vi "Galvo status.vi"() -> ()   [LabVIEW 2018]
uses:
  Controls/ScanType.ctl
  Controls/FGV Actions.ctl
panel:
  out "Scan Type [Out]":T1
  out "Error Out":errorcluster
  in  "Error In":errorcluster
  in  "Actions":T2=enum."Clear"
  out "Status Out":bool
  in  "Status In":bool
  in  "Scan Type [In]":T1
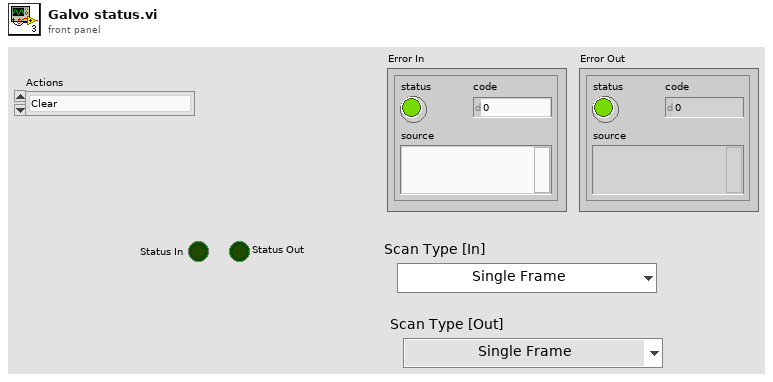
[diagram p1: front panel]
types:
  T1 = typedef "ScanType.ctl" = enum16{"Single Frame", "Continuous Frame", "ROI Line", "Vibratome", "Mosaic", "Mosaic + Slice"}
  T2 = typedef "FGV Actions.ctl" = enum16{"Init", "Set", "Get", "Clear"}
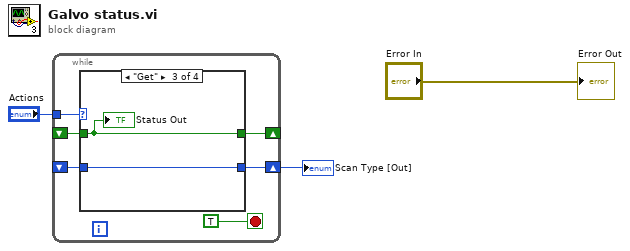
[diagram p0: block diagram]
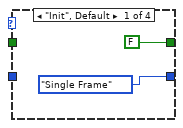
[diagram p2: hidden frame]
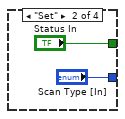
[diagram p3: hidden frame]
diagram:
  n1 = while {
    tunnel: "Actions" -> [w8]
    shift-right: [w7] -> _
    shift-left: _ -> [w6]
    shift-right: [w5] -> w1
    shift-left: _ -> [w4]
    stop <- TRUE stop-if-true
    n2 = case shown="\"Get\"" w8 {
      tunnel: [FALSE "Status In" w15 _] -> w7
      tunnel: w6 -> [_ _ w15 _]
      tunnel: [ScanType."Single Frame" ("Scan Type") "Scan Type [In]" w14 _] -> w5
      tunnel: w4 -> [_ _ w14 _]
      frame "Init", Default {
      }
      frame "Set" {
      }
      frame "Get" {
        "Status Out" <- w15
      }
      frame "Clear" {
      }
    }
  }
  "Scan Type [Out]" <- w1
  "Error Out" <- "Error In"
